vi "Delta T_even_odd.vi"(8 "Background":dbl[][](array[numeric]), 9 "FrameData":dbl[][][](array[numeric])) -> (0 "FrameData even":dbl[][][](array[numeric]), 1 "FrameData odd":dbl[][][](array[numeric]), 2 "Mean even":dbl[][](array[numeric]), 3 "Mean odd":dbl[][](array[numeric]))   [LabVIEW 2020]
uses:
  Random subVIs/Control 1.ctl
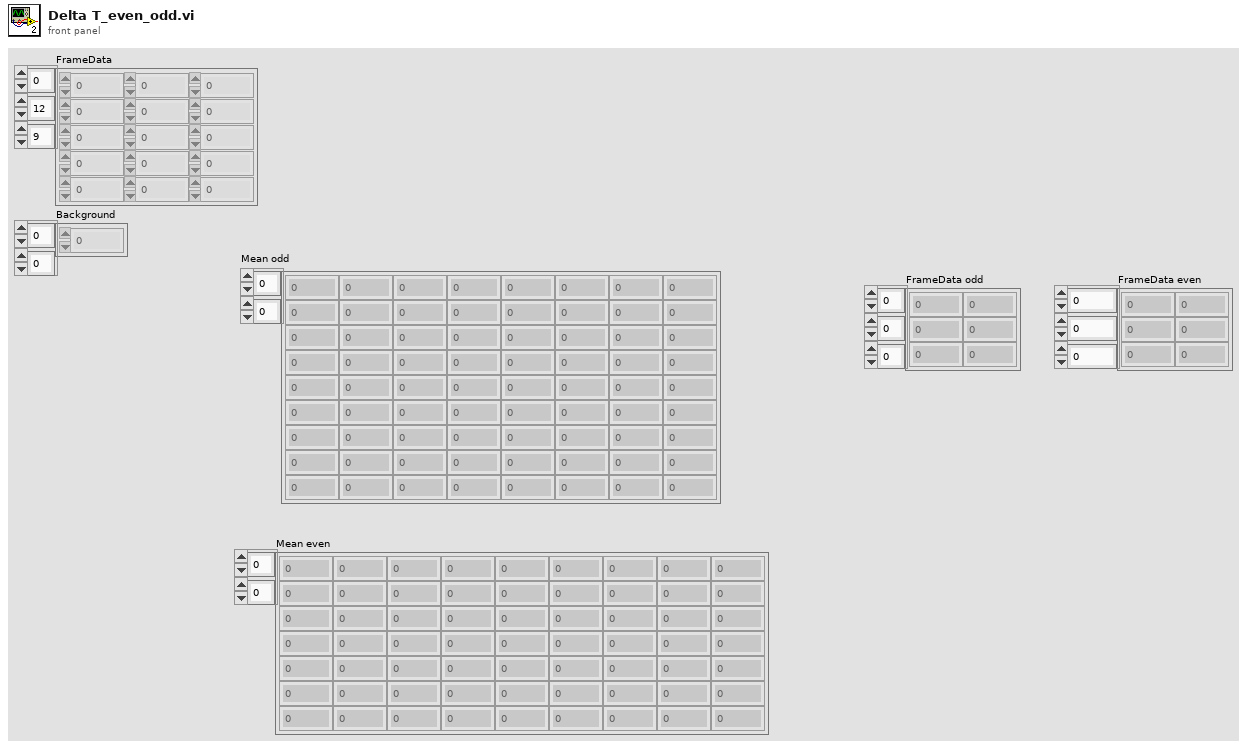
[diagram p1: front panel]
types:
  T1 = typedef "Control 1.ctl" = i32
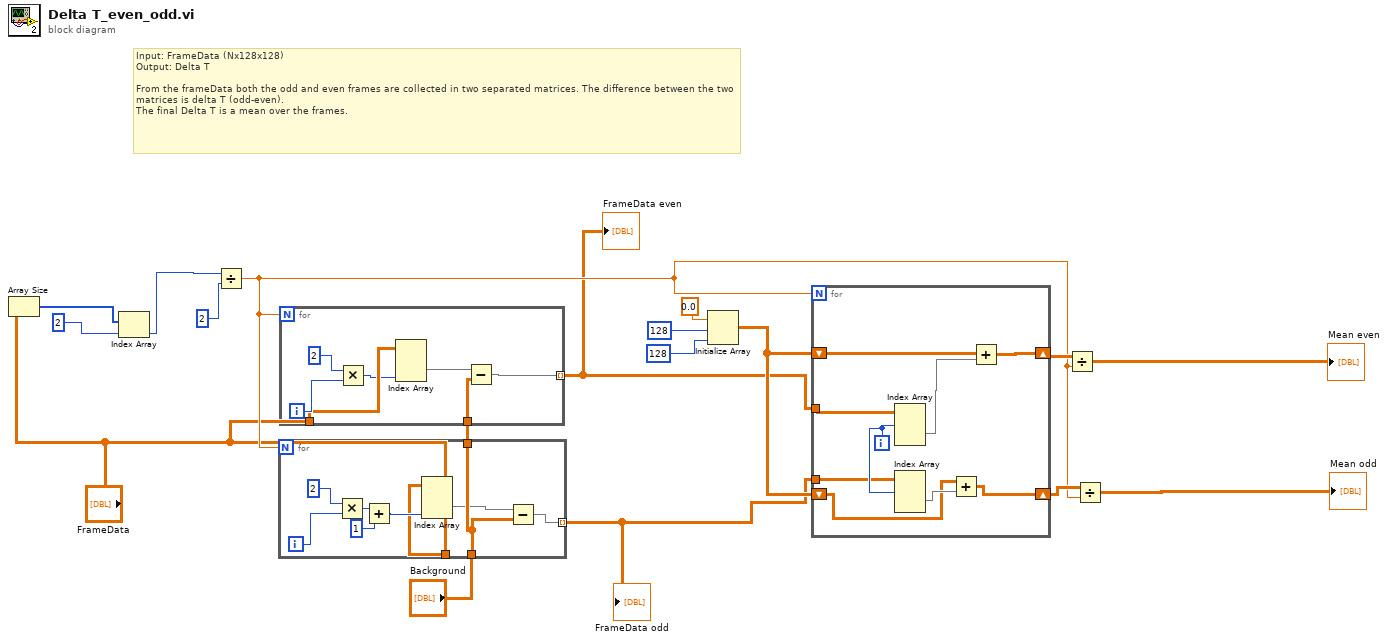
[diagram p0: block diagram]
diagram:
  # "Input: FrameData (Nx128x128)\nOutput: Delta T\n\nFrom the frameData both the odd and even frames are collected in two separated matrices. The difference between the two matrices is delta T (odd-even). \nThe final Delta T is a mean over the frames."
  n1 = Array Size(array="FrameData") -> (size(s)=w12:i32[])
  n2 = Index Array(array=w12, index=2) -> (element=w11:i32)
  n3 = Divide(x=w11, y=T1 2) -> (x/y=w8:dbl)
  n4 = for {
    N: w8 -> [_]
    tunnel: "FrameData" -> [w22]
    tunnel: "Background" -> [w20]
    tunnel: [w21] -> w1 mode=indexing
    tunnel: [w20] -> w6
    i -> [w27]
    n5 = Multiply(x=2, y=w27) -> (x*y=w25:i32)
    n6 = Add(x=w25, y=1) -> (x+y=w23:i32)
    n7 = Index Array(array=w22, index (dim 2)=w23) -> (element=w19:dbl[][])  [unwired: 2 in]
    n8 = Subtract(x=w19, y=w20) -> (x-y=w21:dbl[][])
  }
  "FrameData odd" <- w1
  n9 = for {
    N: w8 -> [_]
    tunnel: [w29] -> w2 mode=indexing
    tunnel: "FrameData" -> [w32]
    tunnel: w6 -> [w30]
    i -> [w34]
    n10 = Multiply(x=2, y=w34) -> (x*y=w31:i32)
    n11 = Index Array(array=w32, index (dim 2)=w31) -> (element=w28:dbl[][])  [unwired: 2 in]
    n12 = Subtract(x=w28, y=w30) -> (x-y=w29:dbl[][])
  }
  "FrameData even" <- w2
  n13 = Initialize Array(0.0 ("element"), 128 ("dimension size"), 128 ("dimension size")) -> (w10:dbl[][])
  n14 = for {
    N: w8 -> [_]
    tunnel: w2 -> [w43]
    shift-right: [w41] -> w14
    shift-left: w10 -> [w36]
    shift-right: [w38] -> w9
    shift-left: w10 -> [w35]
    tunnel: w1 -> [w37]
    i -> [w40]
    n15 = Index Array(array=w43, index (dim 0)=w40) -> (element=w42:dbl[][])  [unwired: 2 in]
    n16 = Index Array(array=w37, index (dim 0)=w40) -> (element=w39:dbl[][])  [unwired: 2 in]
    n17 = Add(x=w35, y=w39) -> (x+y=w38:dbl[][])
    n18 = Add(x=w36, y=w42) -> (x+y=w41:dbl[][])
  }
  n19 = Divide(x=w14, y=w8) -> (x/y=→"Mean even":dbl[][])
  n20 = Divide(x=w9, y=w8) -> (x/y=→"Mean odd":dbl[][])
